vi "Read commandEvents.vi"(8 "error in (no error)":errorcluster, 11 "SAL_Events in":refnum<class "SAL_Events.lvclass">) -> (0 "error out":errorcluster, 2 "commandEvents":T1, 3 "SAL_Events out":refnum<class "SAL_Events.lvclass">)   [LabVIEW 2015, in "SAL_Events.lvclass"]
uses:
  SAL_Events.lvclass
  typedefs/commandsEvents.ctl
  SALLV_dome/DataTypes/command_start.ctl
  SALLV_dome/DataTypes/command_disable.ctl
  SALLV_dome/DataTypes/command_enable.ctl
  SALLV_dome/DataTypes/command_exitControl.ctl
  SALLV_dome/DataTypes/command_standby.ctl
  SALLV_dome/DataTypes/command_stop.ctl
  SALLV_dome/DataTypes/command_Move.ctl
  SALLV_dome/DataTypes/command_Crawl.ctl
  SALLV_dome/DataTypes/command_SetLouvers.ctl
  SALLV_dome/DataTypes/command_Park.ctl
  SALLV_dome/DataTypes/command_StopShutter.ctl
  SALLV_dome/DataTypes/command_OpenShutter.ctl
  SALLV_dome/DataTypes/command_CloseShutter.ctl
  SAL_Events.lvclass/SAL_Events.ctl
  SALLV_dome/SALLV_dome.lvlib
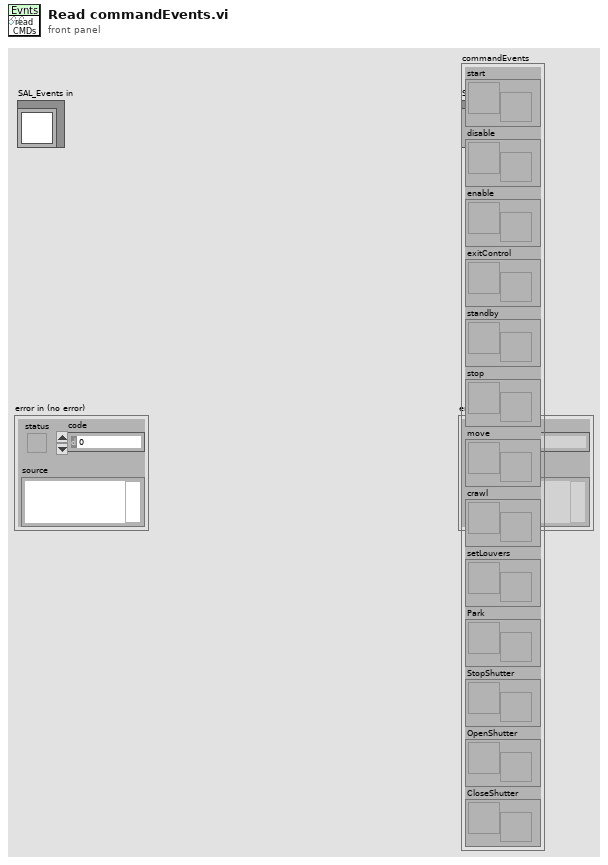
[diagram p1: front panel]
types:
  T1 = typedef "commandsEvents.ctl" = cluster{"start":refnum<user-event>, "disable":refnum<user-event>, "enable":refnum<user-event>, "exitControl":refnum<user-event>, "standby":refnum<user-event>, "stop":refnum<user-event>, "move":refnum<user-event>, "crawl":refnum<user-event>, "setLouvers":refnum<user-event>, "Park":refnum<user-event>, "StopShutter":refnum<user-event>, "OpenShutter":refnum<user-event>, "CloseShutter":refnum<user-event>}
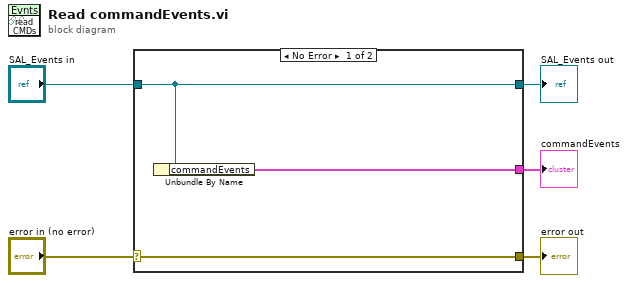
[diagram p0: block diagram]
diagram:
  n1 = case shown="No Error" "error in (no error)" {
    selector: "error in (no error)" -> [w8 w9]
    tunnel: [w8 w9] -> w4
    tunnel: [w7 w10] -> w2
    tunnel: "SAL_Events in" -> [w7 w10]
    tunnel: [w6 _] -> w1
    frame No Error {
      n2 = Unbundle By Name(w7) -> ("commandEvents"=w6:T1)
    }
    frame Error {
    }
  }
  "error out" <- w4
  "SAL_Events out" <- w2
  "commandEvents" <- w1
